vi "Unflatten Asynchronous Execution Units.vi"(8 "error in (no error)":errorcluster, 11 "Compiled Asynchronous Execution Units":T2[](array[typedef])) -> (0 "error out":errorcluster, 3 "Asynchronous Execution Units":T1[](array[typedef]))   [LabVIEW 2020, in "Communication Bus Template Engine.lvlib"]
uses:
  Communication Bus Template Engine.lvlib
  Shared/Asynchronous Execution Unit Compiled Information.ctl
  Asynchronous Execution Unit Runtime Information.ctl
  Includes/Communication Bus Interfaces.lvlibp/Interfaces/Execution Unit/Execution Unit/Execution Unit.lvclass
  Shared/Communication Bus Template Shared.lvlib
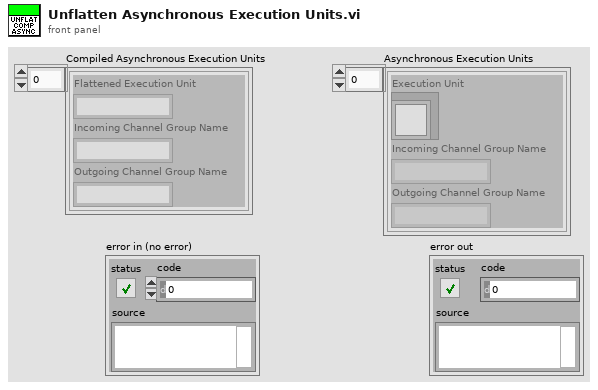
[diagram p1: front panel]
types:
  T1 = typedef "Communication Bus Template Engine.lvlib/Asynchronous Execution Unit Runtime Information.ctl" = cluster{"Execution Unit":refnum<class "Execution Unit.lvclass">, "Incoming Channel Group Name":string, "Outgoing Channel Group Name":string}
  T2 = typedef "Communication Bus Template Shared.lvlib/Asynchronous Execution Unit Compiled Information.ctl" = cluster{"Flattened Execution Unit":string, "Incoming Channel Group Name":string, "Outgoing Channel Group Name":string}
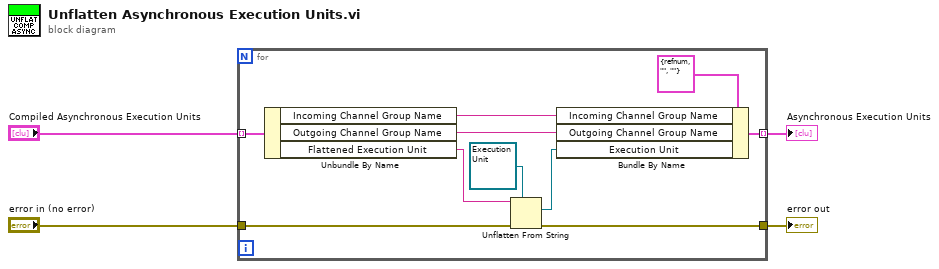
[diagram p0: block diagram]
diagram:
  n1 = for {
    tunnel: "error in (no error)" -> [w14]
    tunnel: [w13] -> w3
    tunnel: "Compiled Asynchronous Execution Units" -> [w11] mode=indexing
    tunnel: [w7] -> w1 mode=indexing
    n2 = Unbundle By Name(w11) -> ("Incoming Channel Group Name"=w6:string, "Outgoing Channel Group Name"=w5:string, "Flattened Execution Unit"=w8:string)
    n3 = Unflatten From String(type=refnum<class "Execution Unit.lvclass"> refnum ("Communication Bus Template Interfaces:Execution Unit.lvlib:Execution Unit.lvclass"), binary string=w8, error in (no error)=w14) -> (value=w9:refnum<class "Execution Unit.lvclass">, error out=w13:errorcluster)  [unwired: 2 in, 1 out]
    n4 = Bundle By Name(cluster=T1 {"Execution Unit"=refnum, "Incoming Channel Group Name"="", "Outgoing Channel Group Name"=""} ("Asynchronous Execution Unit Runtime Information"), "Incoming Channel Group Name"=w6, "Outgoing Channel Group Name"=w5, "Execution Unit"=w9) -> (w7:T1)
  }
  "error out" <- w3
  "Asynchronous Execution Units" <- w1
